vi "Aleator.vi"(2 "minim":dbl, 3 "maxim":dbl) -> (0 "valoare generata":dbl)   [LabVIEW 2025]
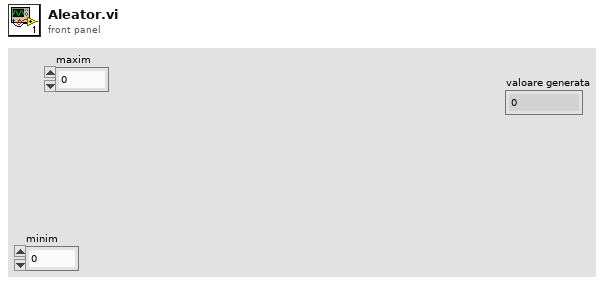
[diagram p1: front panel]
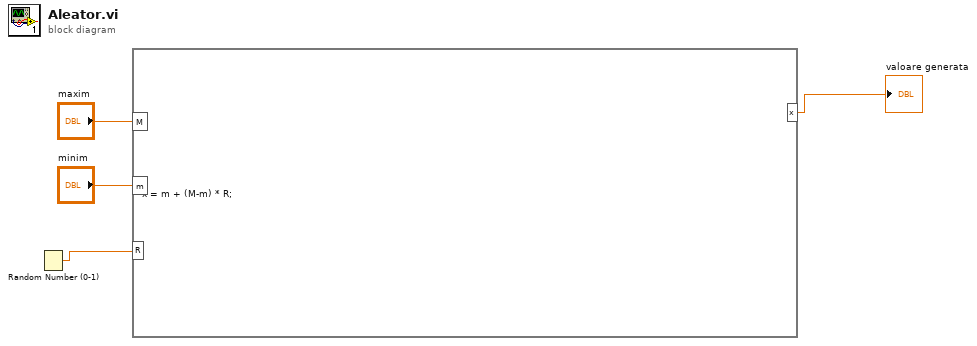
[diagram p0: block diagram]
diagram:
  n1 = Random Number (0-1)() -> (number: 0 to 1=w4:dbl)
  n2 = formula code="x = m + (M-m) * R;"("M"="maxim", "m"="minim", "R"=w4) -> ("x"=→"valoare generata":dbl)
